vi "Set AccessType.vi"(8 "error in":errorcluster, 10 "Value":refnum<class "Value.lvclass">, 11 "Object Type in":refnum<class "Object Type Base.lvclass">) -> (0 "error out":errorcluster, 3 "Object Type out":refnum<class "Object Type Base.lvclass">)   [LabVIEW 2019, in "Electronic Datasheet.lvlib" / "Object Type Base.lvclass"]
uses:
  Object Type Base.lvclass
  Value/Value.lvclass
  Object Type Base.lvclass/Object Type Base.ctl
  Electronic Datasheet.lvlib
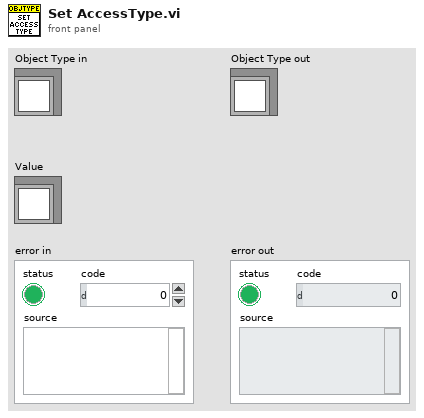
[diagram p1: front panel]
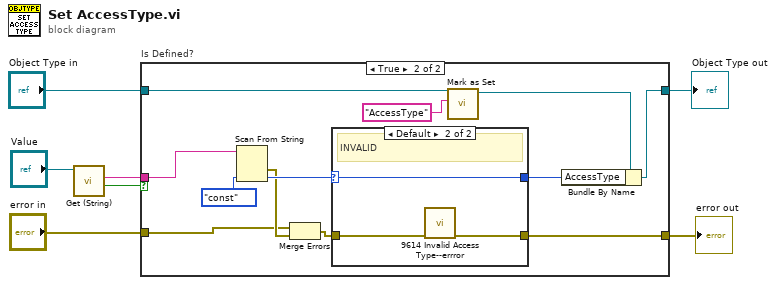
[diagram p0: block diagram]
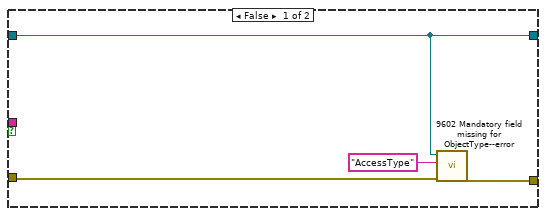
[diagram p2: hidden frame]
diagram:
  n1 = call "Get (String).vi"("Value in"="Value") -> ("Defined?"=w4:bool, "Value"=w3:string)  [unwired: 8 in, 1 out]
  n2 = case "Is Defined?" shown="True" w4 {
    tunnel: [w9 w23] -> w7
    tunnel: "Object Type in" -> [w9 w22]
    tunnel: w3 -> [_ w16]
    tunnel: [w10 w18] -> w2
    tunnel: "error in" -> [w8 w12]
    frame False {
      n3 = call "9602 Mandatory field missing for ObjectType--error.vi"("error in"=w8, "Field Name"="AccessType" ("error message (\"\")"), "Object Type Base"=w9) -> ("error out"=w10:errorcluster)  [unwired: 8 in]
    }
    frame True {
      n4 = Scan From String(input string=w16, default 1=enum16{"ro", "wo", "rw", "rwr", "rww", "const"}."const" ("AccessType")) -> (error out=w14:errorcluster, output 1=w15:enum16{"ro", "wo", "rw", "rwr", "rww", "const"})  [unwired: 3 in, 2 out]
      n5 = Merge Errors(w12, w14) -> (w13:errorcluster)
      n6 = case shown="Default" w15 {
        selector: w15 -> [w25 w27]
        tunnel: [w24 w28] -> w18
        tunnel: [w25 w27] -> w19
        tunnel: w13 -> [w24 w26]
        frame "ro".."const" {
        }
        frame Default {
          # "INVALID"
          n7 = call "9614 Invalid Access Type--errror.vi"("error in"=w26) -> ("error out"=w28:errorcluster)  [unwired: 10 in]
        }
      }
      n8 = call "Mark as Set.vi"("Field name"="AccessType", "Object Type in"=w22) -> ("Object Type out"=w21:refnum<class "Object Type Base.lvclass">)  [unwired: 9 in]
      n9 = Bundle By Name(cluster=w21, "AccessType"=w19) -> (w23:refnum<class "Object Type Base.lvclass">)
    }
  }
  "Object Type out" <- w7
  "error out" <- w2
